vi "serialize_test.vi"() -> ()   [LabVIEW 2016]
uses:
  <vilib>/addons/_JKI.lib/Serialization/JSON/JKI JSON Serialization.lvlib
panel:
  out "X to data?":bool
  out "data to X?":bool
  in  "X":enum16{"JSON", "Flatten"}(ring)
  out "X to data":u32
  out "data to X":u32
  out "data":waveform(dbl)[](array[waveform])
  in  "input signal":waveform(dbl)[](array[waveform])
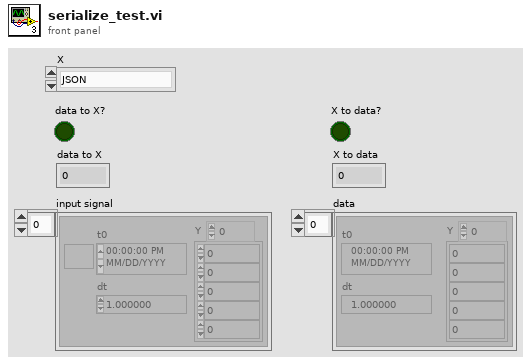
[diagram p1: front panel]
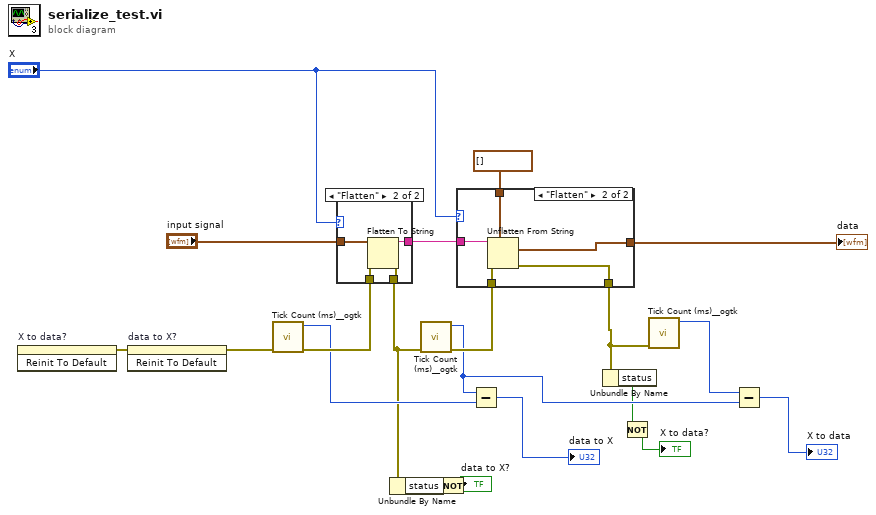
[diagram p0: block diagram]
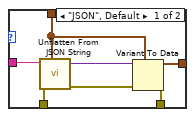
[diagram p2: hidden frame]
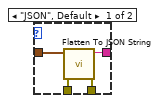
[diagram p3: hidden frame]
diagram:
  n1 = invoke on="X to data?" class="Bool (strict)" method="Reinit To Default"() -> (error out=w4:errorcluster)  [unwired: 3 in, 2 out]
  n2 = invoke on="data to X?" class="Bool (strict)" method="Reinit To Default"(error in=w4) -> (error out=w3:errorcluster)  [unwired: 2 in, 2 out]
  n3 = call <userlib>:"Tick Count (ms)__ogtk.vi"("error in (no error)"=w3) -> ("error out"=w18:errorcluster, "millisecond timer value"=w16:u32)  [unwired: 9 in]
  n4 = case shown="\"Flatten\"" "X" {
    tunnel: [w24 w27] -> w20
    tunnel: [w23 w25] -> w8
    tunnel: w18 -> [w22 w26]
    tunnel: "input signal" -> [w21 w28]
    frame "JSON", Default {
      n5 = call <vilib>:"Flatten To JSON String.vi"("error in (no error)"=w22, "Variant"=w21) -> ("error out"=w23:errorcluster, "JSON String"=w24:string)  [unwired: 8 in]
    }
    frame "Flatten" {
      n6 = Flatten To String(anything=w28, error in (no error)=w26) -> (data string=w27:string, error out=w25:errorcluster)  [unwired: 2 in, 1 out]
    }
  }
  n7 = Unbundle By Name(w8) -> ("status"=w7:bool)
  n8 = call <userlib>:"Tick Count (ms)__ogtk.vi"("error in (no error)"=w8) -> ("error out"=w17:errorcluster, "millisecond timer value"=w11:u32)  [unwired: 9 in]
  n9 = Not(x=w7) -> (.not. x?=→"data to X?":bool)
  n10 = case shown="\"Flatten\"" "X" {
    tunnel: w20 -> [w35 w40]
    tunnel: [w33 w37] -> w19
    tunnel: [w31 w36] -> w6
    tunnel: w17 -> [w30 w39]
    tunnel: waveform(dbl)[] [] ("input signal 2") -> [w29 w38]
    frame "JSON", Default {
      n11 = call <vilib>:"Unflatten From JSON String.vi"("Type and Defaults"=w29, "error in (no error)"=w30, "JSON String"=w35) -> ("error out"=w32:errorcluster, "Variant"=w34:variant)  [unwired: 7 in]
      n12 = Variant To Data(error in=w32, type=w29, Variant=w34) -> (data=w33:waveform(dbl)[], error out=w31:errorcluster)
    }
    frame "Flatten" {
      n13 = Unflatten From String(type=w38, binary string=w40, error in (no error)=w39) -> (value=w37:waveform(dbl)[], error out=w36:errorcluster)  [unwired: 2 in, 1 out]
    }
  }
  "data" <- w19
  n14 = Subtract(x=w11, y=w16) -> (x-y=→"data to X":u32)
  n15 = Unbundle By Name(w6) -> ("status"=w5:bool)
  n16 = Not(x=w5) -> (.not. x?=→"X to data?":bool)
  n17 = call <userlib>:"Tick Count (ms)__ogtk.vi"("error in (no error)"=w6) -> ("millisecond timer value"=w15:u32)  [unwired: 9 in, 1 out]
  n18 = Subtract(x=w15, y=w11) -> (x-y=→"X to data":u32)
